vi "Filter.vi"(10 "log record":T1 {"timestamp" format="%<%x %.3X>T"}, 11 "filter in":refnum<class "Filter.lvclass">) -> (2 "discard?":bool, 3 "filter out":refnum<class "Filter.lvclass">)   [LabVIEW 2018, in "GLog.lvlib" / "Filter.lvclass"]
uses:
  Filter.lvclass
  Log Record.ctl
  logger_class/Internal Log Levels.ctl
  GLog.lvlib
panel:
  # "Connector Pane"
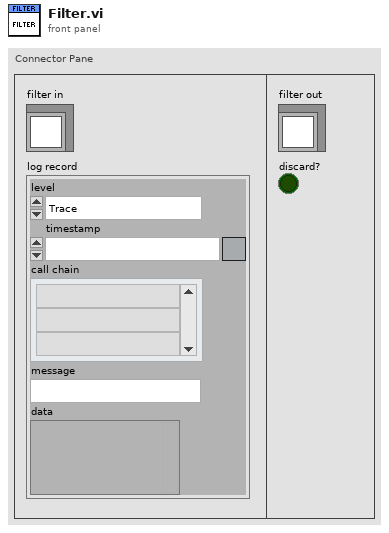
[diagram p1: front panel]
types:
  T1 = typedef "GLog.lvlib/Log Record.ctl" = cluster{"level":T2, "timestamp":timestamp, "call chain":string[], "message":string, "data":variant}
  T2 = typedef "GLog.lvlib/Internal Log Levels.ctl" = enum16{"Trace", "Debug", "Info", "Warning", "Error", "Critical", "Internal"}
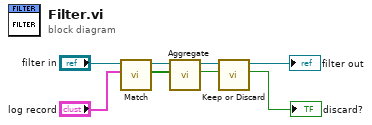
[diagram p0: block diagram]
diagram:
  n1 = call-dynamic "Match.vi"("log record"="log record", "filter in"="filter in") -> ("matches"=w6:bool[], "filter out"=w2:refnum<class "Filter.lvclass">)  [unwired: 8 in]
  n2 = call "Aggregate.vi"("matches"=w6, "filter"=w2) -> ("match?"=w5:bool, "dup filter"=w3:refnum<class "Filter.lvclass">)  [unwired: 8 in]
  n3 = call "Keep or Discard.vi"("match?"=w5, "filter"=w3) -> ("discard?"=→"discard?":bool, "dup filter"=→"filter out":refnum<class "Filter.lvclass">)  [unwired: 8 in]
